vi "System-AsyncUserPlugin.vi"(11 "DSI Reference":refnum<class "DCM-DSI.lvclass">) -> ()   [LabVIEW 2016, in "DSI-RT.lvlib"]
uses:
  DSI-RT.lvlib
  Classes/DCM-DSI/DCM-DSI.lvclass
  <vilib>/Platform/TimedLoop/XDataNode/timing_clust.ctl
  <vilib>/Platform/TimedLoop/XDataNode/nitl_modes.ctl
  <vilib>/Platform/TimedLoop/XDataNode/wakeup.ctl
  Classes/DCM-DSI/Write dt.vi
  Classes/DCM-DSI/Write LoopCount.vi
  <vilib>/Platform/TimedLoop/XDataNode/XDataNode.xnode
  <vilib>/addons/Software Calibration Management/xSCM/CalPoint.xnode
  <vilib>/addons/Software Calibration Management/xSCM/FaultPoint.xnode
  <vilib>/addons/Software Calibration Management/xSCM/ni_scm.dll
  <vilib>/Platform/TimedLoop/XDataNode/XDNodeRunTimeDep.lvlib
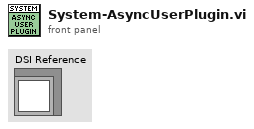
[diagram p1: front panel]
types:
  T1 = typedef "XDNodeRunTimeDep.lvlib/timing_clust.ctl" = cluster{"Expected End [f-1]":u64, "Actual End [f-1]":u64, "Finished Late? [f-1]":bool, "Expected End [i-1]":u64, "Actual End [i-1]":u64, "Finished Late? [i-1]":bool, "Expected Start [i]":u64, "Actual Start [i]":u64, "Expected Start [f]":u64, "Actual Start [f]":u64, "Source Name":string, "Structure Name":string, "Period":i64, "Deadline":i64, "Offset":i64, "Start":i64, "Priority":i32, "Timeout":i32, "Mode":T2, "Wakeup Reason":T3, "Error":errorcluster, "Source Type":string, "Secondary Source Type":string, "Global End Time":u64, "Global Start Time":u64, "Frame Duration":u64, "Iteration Duration":u64, "Assigned CPU":i32, "I/O Scan Engine Mode":u32}
  T2 = typedef "XDNodeRunTimeDep.lvlib/nitl_modes.ctl" = enum32{"No Change", "Process missed periods, maintain original phase", "Discard missed periods, maintain original phase", "Process missed periods, ignore original phase", "Discard missed periods, ignore original phase"}
  T3 = typedef "XDNodeRunTimeDep.lvlib/wakeup.ctl" = enum32{"Normal", "Aborted", "Asynchronous wakeup", "Timing source error", "Timed loop error", "Timeout"}
  T4 = typedef "DSI-Shared.lvlib/UserParameter.ctl" = cluster{"Name":string, "Value":dbl}
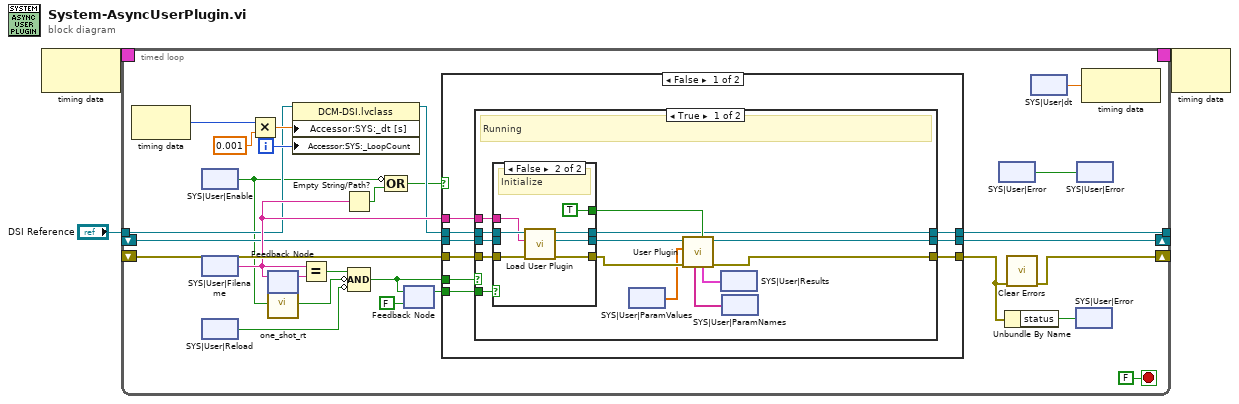
[diagram p0: block diagram]
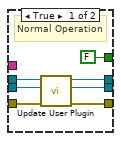
[diagram p2: hidden frame]
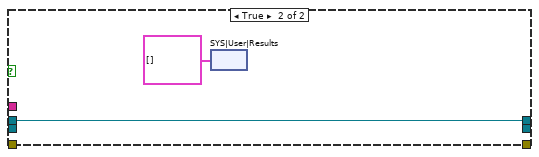
[diagram p4: hidden frame]
diagram:
  n1 = node-c288 ("Input Node")() -> (w2:T1)  [unwired: 1 in]
  n2 = timed-loop {
    shift-right: [w5] -> _
    shift-left: _ -> [w30]
    tunnel: "DSI Reference" -> [w16]
    shift-right: [w20] -> _
    shift-left: _ -> [w14]
    tunnel: [w22] -> _
    timing: w2 -> [_]
    timing-out: [_] -> w1
    i -> [w17]
    stop <- FALSE stop-if-true
    n3 = node-c288 ("Output Node")() -> (w7:i64)  [unwired: 1 in]
    n4 = xnode "SYS|User|Enable"() -> ("Value"=w10:bool)
    n5 = xnode "SYS|User|Filename"() -> ("Value"=w25:string)
    n6 = xnode "SYS|User|Reload"() -> ("Value"=w11:bool)
    n7 = Multiply(x=w7, y=0.001) -> (x*y=w18:sgl)
    n8 = feedback #1() -> (w26:string)  [unwired: 1 in]
    n9 = feedback-in #1(w25) -> ()
    n10 = call <vilib>:"one_shot_rt.vi"("I"=w10) -> ("O"=w9:bool)
    n11 = property class="DCM-DSI.lvclass"(reference=w16, "Accessor:SYS:_dt [s]"=w18, "Accessor:SYS:_LoopCount"=w17) -> (reference out=w15:refnum<class "DCM-DSI.lvclass">)  [unwired: 1 in, 1 out]
    n12 = Equal?(x=w25, y=w26) -> (x = y?=w27:bool)
    n13 = Empty String/Path?(string/path=w25) -> (empty?=w13:bool)
    n14 = Compound Arithmetic op=AND(w27, invert w9, invert w11) -> (w24:bool)
    n15 = Compound Arithmetic op=OR(invert w10, w13) -> (w12:bool)
    n16 = feedback #2(FALSE) -> (w23:bool)
    n17 = feedback-in #2(w24) -> ()
    n18 = case shown="False" w12 {
      tunnel: [w90 w144] -> w22
      tunnel: [w89 _] -> w6
      tunnel: w23 -> [w88 _]
      tunnel: w24 -> [w87 _]
      tunnel: w25 -> [w86 _]
      tunnel: w15 -> [w85 w144]
      tunnel: w30 -> [w84 _]
      tunnel: [w83 _] -> w20
      tunnel: w14 -> [w82 _]
      frame False {
        n19 = case shown="True" w87 {
          tunnel: [w94 w142] -> w90
          tunnel: [w91 _] -> w89
          tunnel: w88 -> [w104 _]
          tunnel: w86 -> [w103 _]
          tunnel: w85 -> [w102 w142]
          tunnel: w84 -> [w101 _]
          tunnel: [w93 _] -> w83
          tunnel: w82 -> [w92 _]
          frame True {
            # "Running"
            n20 = case shown="False" w104 {
              tunnel: [w127 w133] -> w100
              tunnel: [w123 w134] -> w99
              tunnel: w103 -> [_ w130]
              tunnel: w102 -> [w126 w135]
              tunnel: w101 -> [w124 w131]
              tunnel: [FALSE ("Initialize") TRUE ("Initialize")] -> w95
              tunnel: [w125 w132] -> w94
              tunnel: w92 -> [w128 _]
              frame True {
                # "Normal Operation"
                n21 = call "Update User Plugin.vi"("error in (no error)"=w124, "Plugin Reference"=w128, "DSI Reference"=w126) -> ("error out"=w123:errorcluster, "Plugin Reference"=w127:refnum<class "DCM-DSI.lvclass">, "DSI Reference"=w125:refnum<class "DCM-DSI.lvclass">)  [unwired: 6 in]
              }
              frame False {
                # "Initialize"
                n22 = call "Load User Plugin.vi"("error in (no error)"=w131, "Name or relative path"=w130, "DSI Reference"=w135) -> ("error out"=w134:errorcluster, "Plugin Reference"=w133:refnum<class "DCM-DSI.lvclass">, "DSI Reference"=w132:refnum<class "DCM-DSI.lvclass">)  [unwired: 6 in]
              }
            }
            n23 = xnode "SYS|User|ParamValues"() -> ("Value"=w96:sgl[])
            n24 = call-dynamic "User Plugin.vi"("Initialize"=w95, "error in (no error)"=w99, "ParamValues"=w96, "DSI Reference"=w100) -> ("error out"=w91:errorcluster, "DSI Reference"=w93:refnum<class "DCM-DSI.lvclass">, "Results"=w97:T4[], "ParamNames"=w98:string[])  [unwired: 4 in]
            n25 = xnode "SYS|User|Results"("Value"=w97) -> ()
            n26 = xnode "SYS|User|ParamNames"("Value"=w98) -> ()
          }
          frame False {
            # "Off"
          }
        }
      }
      frame True {
        n27 = xnode "SYS|User|Results"("Value"=cluster{"Name":string, "Value":dbl}[] []) -> ()
      }
    }
    n28 = xnode "SYS|User|Error"() -> ("Fault"=w4:bool)
    n29 = Unbundle By Name(w6) -> ("status"=w21:bool)
    n30 = call <vilib>:"Clear Errors.vi"("error in (no error)"=w6) -> ("error out"=w5:errorcluster)  [unwired: 5 in, 1 out]
    n31 = xnode "SYS|User|dt"() -> ("Value"=w8:sgl)
    n32 = xnode "SYS|User|Error"("Fault"=w21) -> ()
    n33 = xnode "SYS|User|Error"("Value"=w4) -> ()
    n34 = node-c288 ("Input Node")(w8) -> ()  [unwired: 1 out]
  }
  n35 = node-c288 ("Output Node")(w1) -> ()  [unwired: 1 out]
